vi "SubVI Terminals Duplicate.vi"(6 "Label":string, 8 "error in":errorcluster, 10 "VI":refnum<vi>) -> (0 "error out":errorcluster, 2 "Terminals[]":refnum<vi>[](array[refnum]))   [LabVIEW 2025, in "_Rescript.lvlib"]
uses:
  _Rescript.lvlib
  <vilib>/Utility/traverseref.llb/TRef TravTarget.ctl
  <vilib>/Utility/traverseref.llb/VI Scripting - Traverse.lvlib
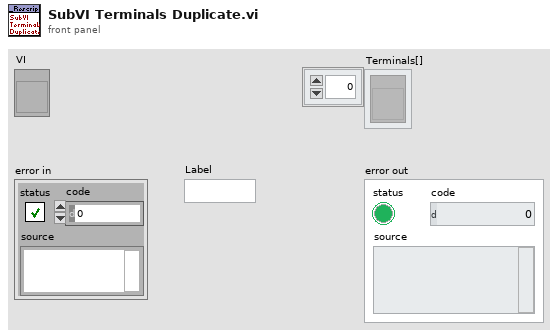
[diagram p1: front panel]
types:
  T1 = typedef "TRef TravTarget.ctl" = enum16{"FP", "BD", "Other"}
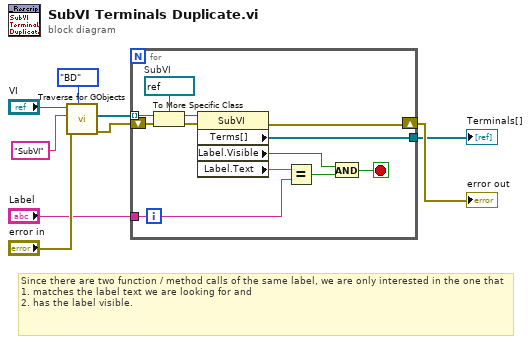
[diagram p0: block diagram]
diagram:
  # "Since there are two function / method calls of the same label, we are only interested in the one that\n1. matches the label text we are looking for and\n2. has the label visible."
  n1 = call <vilib>:"Traverse for GObjects.vi"("Traverse Target"=TRef_TravTarget."BD", "error in (no error)"="error in", "Class Name"="SubVI", "VI Refnum"="VI") -> ("error out"=w4:errorcluster, "References"=w5:refnum<vi>[])  [unwired: 4 in, 2 out]
  n2 = for {
    tunnel: w5 -> [w20] mode=indexing
    tunnel: "Label" -> [w17]
    tunnel: [w14] -> w1
    shift-right: [w13] -> w2
    shift-left: w4 -> [w19]
    stop <- w16 stop-if-true
    w21 = refnum<vi> refnum  # SubVI
    n3 = To More Specific Class(target class=w21, reference=w20, error in=w19) -> (specific class reference=w18:refnum<vi>, error out=w15:errorcluster)
    n4 = property class="SubVI"(reference=w18, error in=w15) -> (error out=w13:errorcluster, "Terms[]"=w14:refnum<vi>[], "Label.Visible"=w12:bool, "Label.Text"=w11:string)  [unwired: 1 out]
    n5 = Equal?(x=w11, y=w17) -> (x = y?=w10:bool)
    n6 = And(x=w12, y=w10) -> (x .and. y?=w16:bool)
  }
  "error out" <- w2
  "Terminals[]" <- w1
